vi "Preferences Keys.vi"() -> ()   [LabVIEW 2018, in "Bookmark Manager.lvlib"]
uses:
  Bookmark Manager.lvlib
panel:
  in  "Show Resource VIs":string="Eulogy.Graveyard.Position"
  in  "Show vi.libs VIs":string="Eulogy.Graveyard.Position"
  in  "Column Resizing Key":string="Eulogy.Graveyard.Position"
  in  "Window Size Key":string="Eulogy.Graveyard.Position"
  in  "Grouping Key":string
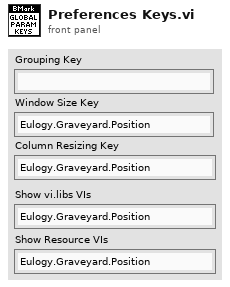
[diagram p1: front panel]
diagram:
